vi "FPGA_CounterOpen WO Configuration.vi"(8 "error in":errorcluster, 11 "CntIndex":T1) -> (0 "error out":errorcluster, 3 "Ctr Ref":T2)   [LabVIEW 2017]
uses:
  <vilib>/Rock Robotics/SystemInterfaces/Counter/FPGA_CounterCtrDevRef.ctl
  <vilib>/Rock Robotics/SystemInterfaces/Counter/FPGA_CounterCtrSystemIndex.ctl
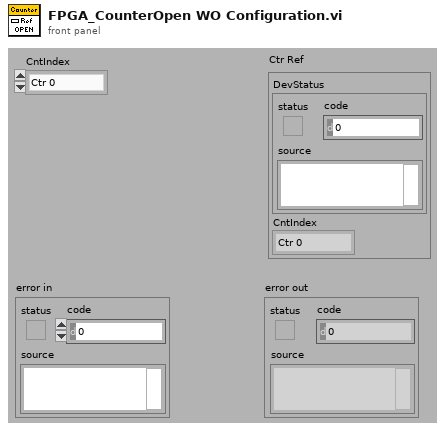
[diagram p1: front panel]
types:
  T1 = typedef "FPGA_CounterCtrSystemIndex.ctl" = enum8{"Ctr 0", "Ctr 1", "Ctr 2", "Ctr 3", "Ctr 4", "Ctr 5", "Ctr 6", "Ctr 7", "Invalid"}
  T2 = typedef "FPGA_CounterCtrDevRef.ctl" = cluster{"DevStatus":errorcluster, "CntIndex":T1}
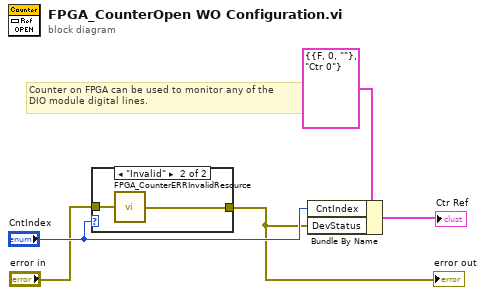
[diagram p0: block diagram]
diagram:
  # "Counter on FPGA can be used to monitor any of the \nDIO module digital lines."
  n1 = case shown="\"Invalid\"" "CntIndex" {
    tunnel: [w6 w8] -> w3
    tunnel: "error in" -> [w6 w7]
    frame Default {
    }
    frame "Invalid" {
      n2 = call <vilib>:"FPGA_CounterERRInvalidResource.vi"("error in (no error)"=w7) -> ("error out"=w8:errorcluster)
    }
  }
  "error out" <- w3
  n3 = Bundle By Name(cluster=T2 {"DevStatus"={"status"=FALSE, "code"=0, "source"=""}, "CntIndex"=enum."Ctr 0"} ("Ctr Ref"), "CntIndex"="CntIndex", "DevStatus"=w3) -> (→"Ctr Ref":T2)
